vi "update_dust_event.vi"   [LabVIEW 2013]
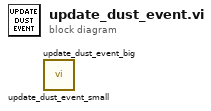
[diagram p0: block diagram]
diagram:
  n1 = call "update_dust_event_small.vi"() -> ()  [unwired: 11 in, 1 out]
  n2 = call "update_dust_event_big.vi"() -> ()  [unwired: 11 in, 1 out]
